vi "car_config.vi"() -> (1 "Torque/MPH":cluster{dbl[], dbl[]}[](graph), 2 "RPM/MPH":cluster{dbl[], "all rows":dbl[]}[](graph))   [LabVIEW 2025]
panel:
  in  "Wheel Diameter":i32=16
  in  "Sidewall %":i32=50
  in  "Tyre width":i32=195
  in  "Torque/RPM":dbl[][](array[numeric])=[[1000.0, 49.0], [1500.0, 73.0], [2000.0, 85.0], [2500.0, 93.0], [3000.0, 98.0], [3500.0, 101.0], [4000.0, 104.0], [4500.0, 105.0], [5000.0, 103.0], [5500.0, 99.0], [6000.0, 91.0], [6500.0, 76.0]]
  in  "Gear Ratios":dbl[][](array[numeric])=[[14.0, 61.0], [11.0, 41.0], [21.0, 43.0], [28.0, 39.0], [31.0, 34.0], [37.0, 33.0]]
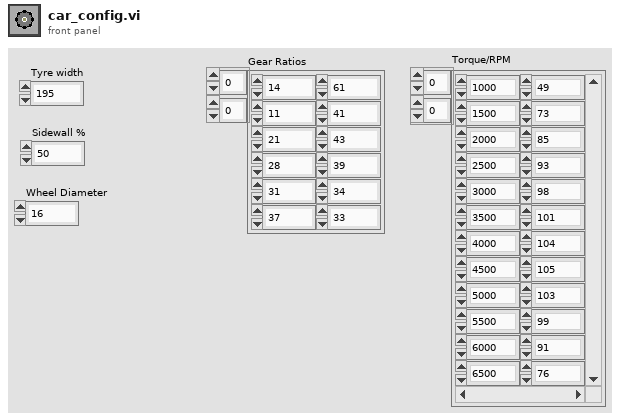
[diagram p1: front panel]
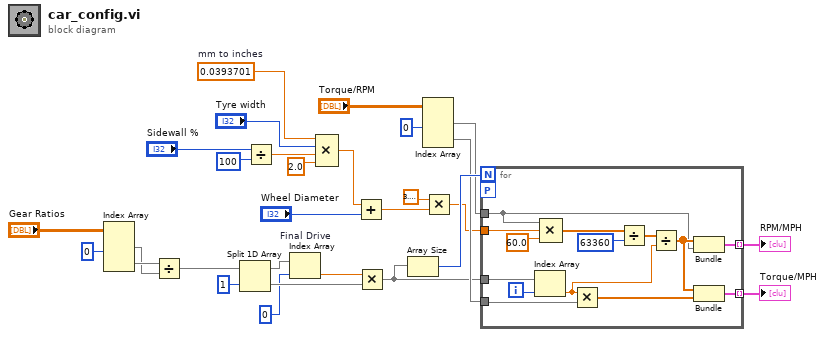
[diagram p0: block diagram]
diagram:
  w1 = 0.0393701  # mm to inches
  n1 = Index Array(array="Gear Ratios", index (col) #1=0 ("index (col)")) -> (element #1=w27:dbl[], element #2=w28:dbl[])  [unwired: 3 in]
  n2 = Divide(x=w28, y=w27) -> (x/y=w21:dbl[])
  n3 = Split 1D Array(array=w21, index=1) -> (first subarray=w23:dbl[], second subarray=w25:dbl[])
  n4 = Divide(x="Sidewall %", y=100) -> (x/y=w3:dbl)
  n5 = Index Array "Final Drive"(array=w23, index=0) -> (element=w26:dbl)
  n6 = Compound Arithmetic op=MULTIPLY(w1, "Tyre width", w3, 2.0 ("y")) -> (w4:dbl)
  n7 = Add(x=w4, y="Wheel Diameter") -> (x+y=w16:dbl)
  n8 = Multiply(x=w26, y=w25) -> (x*y=w8:dbl[])
  n9 = Array Size(array=w8) -> (size(s)=w14:i32)
  n10 = Index Array(array="Torque/RPM", index (col) #1=0 ("index (col)")) -> (element #1=w10:dbl[], element #2=w9:dbl[])  [unwired: 3 in]
  n11 = Multiply(x=3.141592653589793 ("Pi"), y=w16) -> (x*y=w6:dbl)
  n12 = for {
    N: w14 -> [_]
    tunnel: w8 -> [w42]
    tunnel: w9 -> [w36]
    tunnel: w10 -> [w32]
    tunnel: [w40] -> w12 mode=indexing
    tunnel: [w35] -> w13 mode=indexing
    tunnel: w6 -> [w31]
    workers-P: _ -> [_]
    i -> [w43]
    n13 = Index Array(array=w42, index=w43) -> (element=w34:dbl)
    n14 = Compound Arithmetic op=MULTIPLY(w32, w31, 60.0 ("y")) -> (w30:dbl[])
    n15 = Multiply(x=w34, y=w36) -> (x*y=w41:dbl[])
    n16 = Divide(x=w30, y=63360) -> (x/y=w39:dbl[])
    n17 = Divide(x=w39, y=w34) -> (x/y=w37:dbl[])
    n18 = Bundle(w37, "Torque/RPM"=w32) -> (w35:cluster{dbl[], "Torque/RPM":dbl[]})  [unwired: 1 in]
    n19 = Bundle(w37, w41) -> (w40:cluster{dbl[], dbl[]})  [unwired: 1 in]
  }
  "Torque/MPH" <- w12
  "RPM/MPH" <- w13
